vi "Launcher.vi"   [LabVIEW 2019]
uses:
  GUI_Actor/GUI_Actor.lvclass
  C:/Program Files/National Instruments/LabVIEW 2019/vi.lib/ActorFramework/Actor/Actor.lvclass
  <vilib>/ActorFramework/Actor/Actor.lvclass
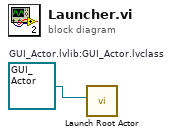
[diagram p0: block diagram]
diagram:
  w1 = refnum<class "GUI_Actor.lvclass"> refnum  # GUI_Actor.lvlib:GUI_Actor.lvclass
  n1 = call <vilib>:"Launch Root Actor.vi"("Actor"=w1) -> ()  [unwired: 9 in, 2 out]
